vi "Initialize.vi"(8 "error in (no error)":errorcluster, 11 "Delta Robot Kinematics":refnum<class "Delta Robot Kinematics.lvclass">) -> (0 "error out":errorcluster, 3 "Delta Analyzor out":refnum<class "Delta Analyzor.lvclass">)   [LabVIEW 2014, in "Delta Analyzor.lvclass"]
uses:
  Delta Analyzor.lvclass
  Delta Robot Kinematics/Delta Robot Kinematics.lvclass
  Delta Analyzor.lvclass/Delta Analyzor.ctl
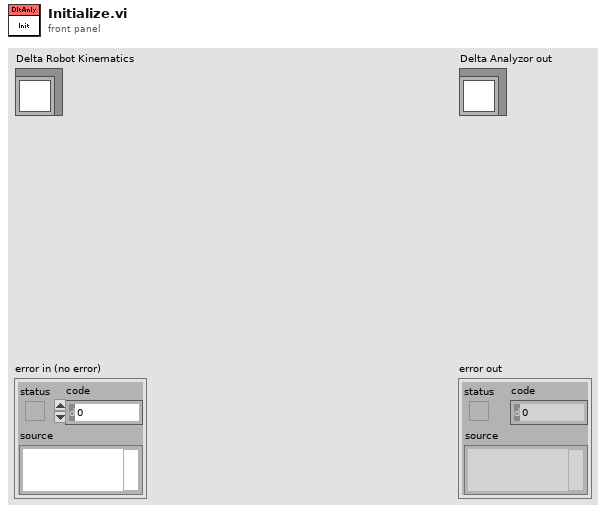
[diagram p1: front panel]
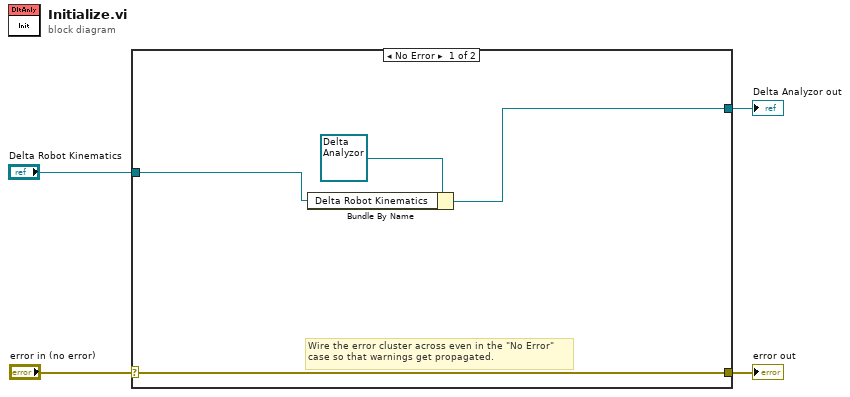
[diagram p0: block diagram]
diagram:
  n1 = case shown="No Error" "error in (no error)" {
    selector: "error in (no error)" -> [w8 w9]
    tunnel: [w8 w9] -> w3
    tunnel: [w5 _] -> w2
    tunnel: "Delta Robot Kinematics" -> [w6 _]
    frame No Error {
      # "Wire the error cluster across even in the \"No Error\"\ncase so that warnings get propagated."
      n2 = Bundle By Name(cluster=refnum<class "Delta Analyzor.lvclass"> refnum ("Delta Analyzor.lvclass"), "Delta Robot Kinematics"=w6) -> (w5:refnum<class "Delta Analyzor.lvclass">)
    }
    frame Error {
    }
  }
  "error out" <- w3
  "Delta Analyzor out" <- w2
